vi "Init REQ Socket.vi"(8 "error in (no error)":errorcluster, 9 "ZMQ new Timeouts in":T1={"SNDTIMEO"=-1, "RCVTIMEO"=-1}, 11 "endpoint":string) -> (0 "error out":errorcluster, 1 "ZMQ new Timeouts out":T1, 2 "socket out":refnum<class "zmq_socket.lvclass">, 3 "zmq_context out":refnum<class "zmq_context.lvclass">)   [LabVIEW 2018, in "LV2Julia_core.lvlib"]
uses:
  LV2Julia_core.lvlib
  <vilib>/addons/zeromq/zmq_context.lvclass
  <vilib>/addons/zeromq/zmq_socket.lvclass
  ZMQ timeouts.ctl
  <vilib>/addons/zeromq/socket_type.ctl
  <vilib>/addons/zeromq/zeromq.lvlib
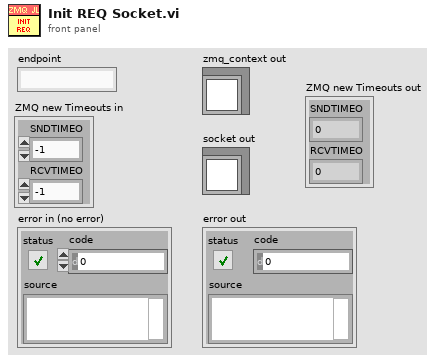
[diagram p1: front panel]
types:
  T1 = typedef "LV2Julia_core.lvlib/ZMQ timeouts.ctl" = cluster{"SNDTIMEO":i32, "RCVTIMEO":i32}
  T2 = typedef "zeromq.lvlib/socket_type.ctl" = enum8{"ZMQ_PAIR", "ZMQ_PUB", "ZMQ_SUB", "ZMQ_REQ", "ZMQ_REP", "ZMQ_DEALER", "ZMQ_ROUTER", "ZMQ_PULL", "ZMQ_PUSH", "ZMQ_XPUB", "ZMQ_XSUB"}
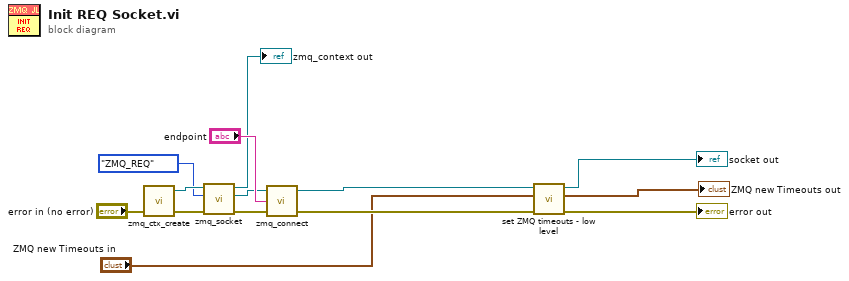
[diagram p0: block diagram]
diagram:
  n1 = call <vilib>:"zmq_ctx_create.vi"("error in"="error in (no error)") -> ("error out"=w10:errorcluster, "context out"=w11:refnum<class "zmq_context.lvclass">)  [unwired: 3 in]
  n2 = call <vilib>:"zmq_socket.vi"("error in"=w10, "socket type"=socket_type."ZMQ_REQ", "context in"=w11) -> ("error out"=w8:errorcluster, "socket out"=w7:refnum<class "zmq_socket.lvclass">, "context out"=→"zmq_context out":refnum<class "zmq_context.lvclass">)  [unwired: 2 in]
  n3 = call <vilib>:"zmq_connect.vi"("error in"=w8, "endpoint"="endpoint", "socket in"=w7) -> ("error out"=w6:errorcluster, "socket out"=w4:refnum<class "zmq_socket.lvclass">)  [unwired: 1 in]
  n4 = call "set ZMQ timeouts - low level.vi"("error in (no error)"=w6, "ZMQ new Timeouts in"="ZMQ new Timeouts in", "zmq_socket in"=w4) -> ("error out"=→"error out":errorcluster, "ZMQ new Timeouts out"=→"ZMQ new Timeouts out":T1, "zmq_socket out"=→"socket out":refnum<class "zmq_socket.lvclass">)  [unwired: 6 in]
